vi "PathPlanner_GridPos_FromJSON.vi"(11 "JSON String":string) -> (0 "Error":bool, 3 "PathPlanner_Grid":T1 {"Field Size M"."Y" format="%14.3f"; "Field Size M"."X" format="%14.3f"})   [LabVIEW 2019, in "PathPlanner24.lvlib"]
doc: "Load a path from a JSON string.\n\nInputs: \n - JSON String - string- The string containing the path definition.\n\nOutputs:\n - Path - cluster - PathPlannerPath created from the given JSON string\n - Error out - cluster - Error cluster"
uses:
  PathPlanner24.lvlib
  TypeDef/PathPlannerGrid.ctl
  <vilib>/Rock Robotics/WPI/ThirdParty/JAS_Junk/TrajLib/TypeDef/TRANSLATION2D.ctl
  <vilib>/Rock Robotics/WPI/ThirdParty/JAS_Junk/TrajLib/Trajectory_Library.lvlib
panel:
  in  "field_size":cluster{"x":dbl, "height":dbl}
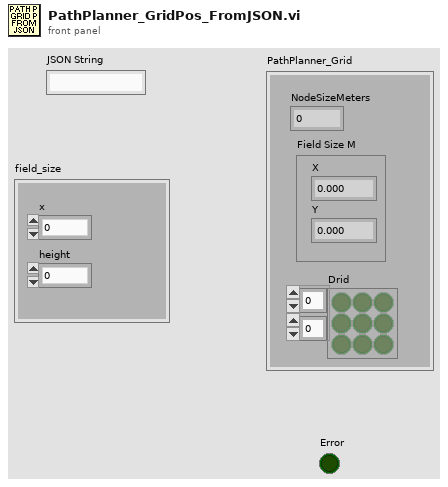
[diagram p1: front panel]
types:
  T1 = typedef "PathPlanner24.lvlib/PathPlannerGrid.ctl" = cluster{"NodeSizeMeters":dbl, "Field Size M":T2, "Drid":bool[][]}
  T2 = typedef "Trajectory_Library.lvlib/TRANSLATION2D.ctl" = cluster{"X":dbl, "Y":dbl}
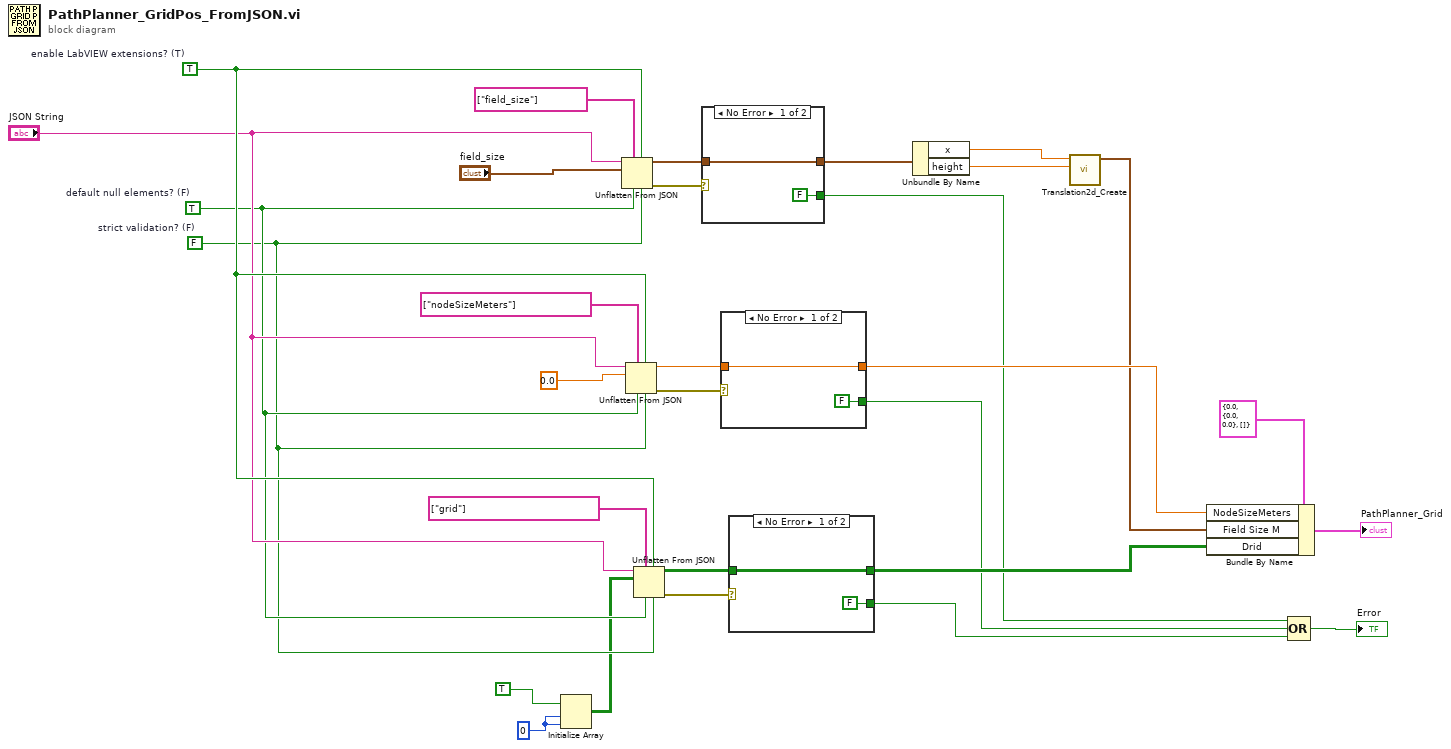
[diagram p0: block diagram]
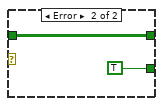
[diagram p2: hidden frame]
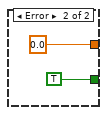
[diagram p3: hidden frame]
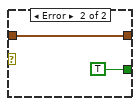
[diagram p4: hidden frame]
diagram:
  w15 = 0 ("dimension size")
  w16 = FALSE  # strict validation? (F)
  w17 = TRUE  # default null elements? (F)
  w19 = TRUE  # enable LabVIEW extensions? (T)
  n1 = Initialize Array(TRUE, w15, w15) -> (w14:bool[][])
  n2 = Unflatten From JSON(path=string[] ["field_size"] ("path 3"), enable LabVIEW extensions? (T)=w19, JSON string="JSON String", type and defaults="field_size", default null elements? (F)=w17, strict validation? (F)=w16) -> (value=w27:cluster{"x":dbl, "height":dbl}, error out=w28:errorcluster)  [unwired: 1 in]
  n3 = Unflatten From JSON(path=string[] ["nodeSizeMeters"] ("path 3"), enable LabVIEW extensions? (T)=w19, JSON string="JSON String", type and defaults=0.0, default null elements? (F)=w17, strict validation? (F)=w16) -> (value=w25:dbl, error out=w26:errorcluster)  [unwired: 1 in]
  n4 = Unflatten From JSON(path=string[] ["grid"] ("path 3"), enable LabVIEW extensions? (T)=w19, JSON string="JSON String", type and defaults=w14, default null elements? (F)=w17, strict validation? (F)=w16) -> (value=w20:bool[][], error out=w21:errorcluster)  [unwired: 1 in]
  n5 = case shown="No Error" w28 {
    tunnel: w27 -> [w32 w34]
    tunnel: [w32 w34] -> w9
    tunnel: [FALSE TRUE] -> w3
    frame No Error {
    }
    frame Error {
    }
  }
  n6 = case shown="No Error" w26 {
    tunnel: w25 -> [w36 _]
    tunnel: [w36 0.0] -> w10
    tunnel: [FALSE TRUE] -> w2
    frame No Error {
    }
    frame Error {
    }
  }
  n7 = case shown="No Error" w21 {
    tunnel: w20 -> [w40 w42]
    tunnel: [w40 w42] -> w5
    tunnel: [FALSE TRUE] -> w4
    frame No Error {
    }
    frame Error {
    }
  }
  n8 = Unbundle By Name(w9) -> ("x"=w8:dbl, "height"=w7:dbl)
  n9 = call <vilib>:"Translation2d_Create.vi"("Y"=w7, "X"=w8) -> ("TRANSLATION"=w6:T2)  [unwired: 9 in]
  n10 = Bundle By Name(cluster=T1 {"NodeSizeMeters"=0.0, "Field Size M"={"X"=0.0, "Y"=0.0}, "Drid"=[]} ("PathPlanner_Grid"), "NodeSizeMeters"=w10, "Field Size M"=w6, "Drid"=w5) -> (→"PathPlanner_Grid":T1)
  n11 = Compound Arithmetic op=OR(w3, w2, w4) -> (→"Error":bool)
